vi "Read Both Fans Fault and State.vi"(8 "error in (no error)":cluster{"状态":bool, "代码":i32, "源":string} caption="错误输入（无错误）", 11 "仿真双风扇输入":refnum<class "Simulated Dual Fan.lvclass">) -> (0 "error out":cluster{"状态":bool, "代码":i32, "源":string} caption="错误输出", 1 "风扇B故障":bool, 2 "风扇B状态":bool, 3 "风扇A故障":bool, 5 "风扇A状态":bool)   [LabVIEW 2015, in "Simulated Dual Fan.lvclass"]
uses:
  Simulated Dual Fan.lvclass
  Cooler Plug-Ins/Simulated Evaporative Cooler.lvclass/Simulation Data_Global.vi
  Cooler Plug-Ins/Simulated Evaporative Cooler.lvclass/Simulated Evaporative Cooler.lvclass
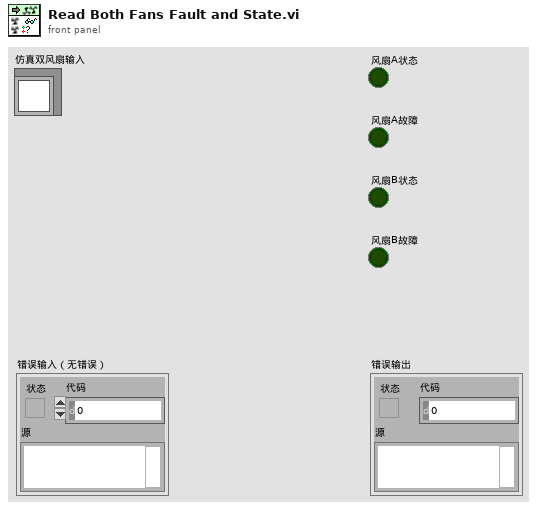
[diagram p1: front panel]
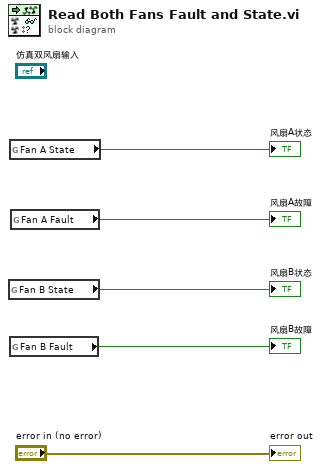
[diagram p0: block diagram]
diagram:
  n1 = global read "Simulation Data_Global.vi" "Fan B State"() -> (→"风扇B状态":bool)
  n2 = global read "Simulation Data_Global.vi" "Fan A State"() -> (→"风扇A状态":bool)
  n3 = global read "Simulation Data_Global.vi" "Fan B Fault"() -> (→"风扇B故障":bool)
  n4 = global read "Simulation Data_Global.vi" "Fan A Fault"() -> (→"风扇A故障":bool)
  "error out" <- "error in (no error)"
